vi "Write Config.vi"(8 "error in (no error)":errorcluster, 10 "Config":variant, 11 "CsvReportPlugin in":refnum<class "CsvReportPlugin.lvclass">) -> (0 "error out":errorcluster, 3 "CsvReportPlugin out":refnum<class "CsvReportPlugin.lvclass">)   [LabVIEW 2015, in "CsvReportPlugin.lvclass"]
uses:
  CsvReportPlugin.lvclass
  CsvReportPlugin.lvclass/CsvReportPlugin.ctl
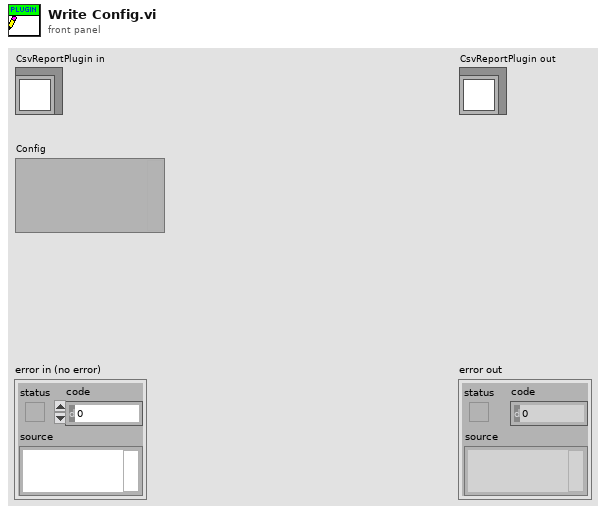
[diagram p1: front panel]
types:
  T1 = cluster{"Enable":bool, "Report Folder":string, "Skip Error Result":bool}
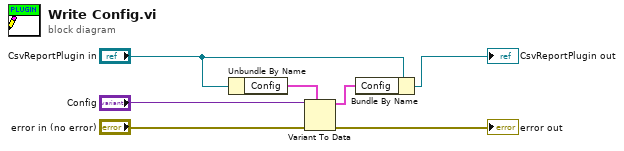
[diagram p0: block diagram]
diagram:
  n1 = Unbundle By Name("CsvReportPlugin in") -> ("Config"=w7:T1)
  n2 = Variant To Data(error in="error in (no error)", type=w7, Variant="Config") -> (data=w6:T1, error out=→"error out":errorcluster)
  n3 = Bundle By Name(cluster="CsvReportPlugin in", "Config"=w6) -> (→"CsvReportPlugin out":refnum<class "CsvReportPlugin.lvclass">)
